vi "SRS865A--read--V1.vi"(8 "error in (no error)":errorcluster, 11 "VISA resource name":refnum<visa-resource-name>) -> (0 "error out":errorcluster, 1 "freq out":dbl, 2 "zi out (V)":cdb, 3 "VISA resource name out":refnum<visa-resource-name>)   [LabVIEW 2017]
uses:
  <instrlib>/Stanford Research SR865/Stanford Research SR865.lvlib
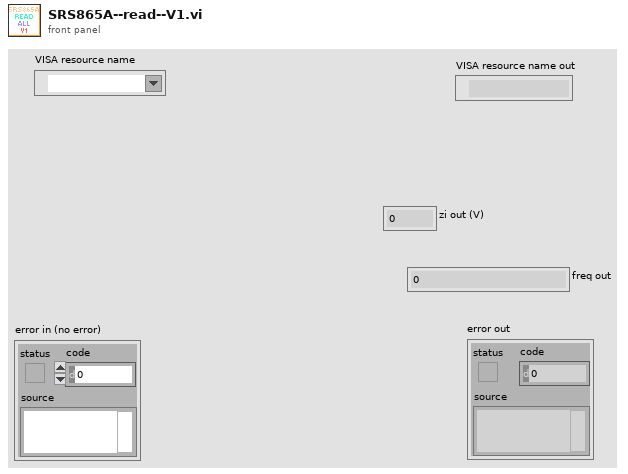
[diagram p1: front panel]
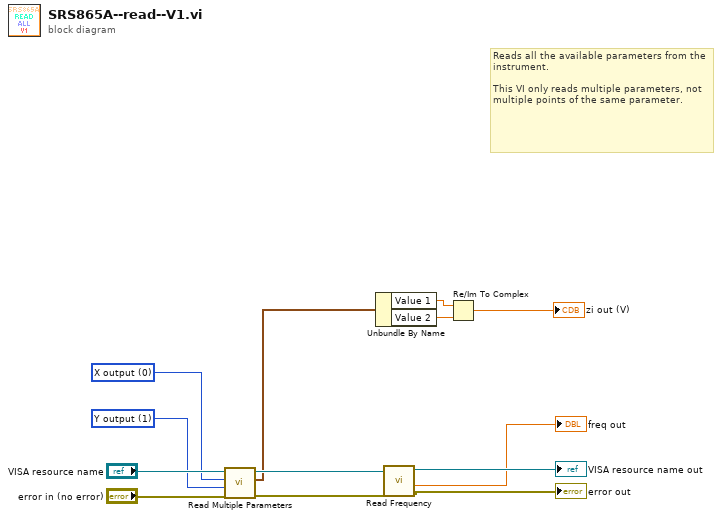
[diagram p0: block diagram]
diagram:
  w7 = 1 items=["X output", "Y output", "R output", "Theta output", "Aux In 1", "Aux In 2", "Aux In 3", "Aux In 4", "Aux Out 1", "Aux Out 2", "Xnoise", "Ynoise", "Reference Phase", "Sine Out Amplitude", "DC Level", "Int. Ref. Frequency", "Ext. Ref. Frequency"] ("Single Lock-in Parameter 2 (0: X output)")
  w6 = 0 items=["X output", "Y output", "R output", "Theta output", "Aux In 1", "Aux In 2", "Aux In 3", "Aux In 4", "Aux Out 1", "Aux Out 2", "Xnoise", "Ynoise", "Reference Phase", "Sine Out Amplitude", "DC Level", "Int. Ref. Frequency", "Ext. Ref. Frequency"] ("Single Lock-in Parameter 1 (0: X output)")
  # "Reads all the available parameters from the instrument.\n\nThis VI only reads multiple parameters, not multiple points of the same parameter."
  n1 = call <instrlib>:"Read Multiple Parameters.vi"("error in (no error)"="error in (no error)", "Single Lock-in Parameter 2 (0: X output)"=w7, "Single Lock-in Parameter 1 (0: X output)"=w6, "VISA resource name"="VISA resource name") -> ("error out"=w9:errorcluster, "Output Value(2 parameters)"=w5:cluster{"Value 1":dbl, "Value 2":dbl}, "VISA resource name out"=w12:refnum<visa-resource-name>)  [unwired: 4 in, 1 out]
  n2 = Unbundle By Name(w5) -> ("Value 1"=w3:dbl, "Value 2"=w4:dbl)
  n3 = call <instrlib>:"Read Frequency.vi"("error in (no error)"=w9, "VISA resource name"=w12) -> ("error out"=→"error out":errorcluster, "Detection Frequency"=→"freq out":dbl, "VISA resource name out"=→"VISA resource name out":refnum<visa-resource-name>)  [unwired: 6 in, 1 out]
  n4 = Re/Im To Complex(1:w4, 2:w3) -> (0:→"zi out (V)":cdb)
